vi "DOTNET - Network Ping v2.0.vi"(0 "IP/Address":string="127.0.0.1", 5 "SetSize":i32=32, 7 "timeout":i32=100, 11 "error in (no error)":errorcluster) -> (4 "Status":i32(ring) items=["Success"=0, "DestinationNetworkUnreachable"=11002, "DestinationHostUnreachable"=11003, "DestinationProhibited, DestinationProtocolUnreachable"=11004, "DestinationPortUnreachable"=11005, "NoResources"=11006, "BadOption"=11007, "HardwareError"=11008, "PacketTooBig"=11009, "TimedOut"=11010, "BadRoute"=11012, "TtlExpired"=11013, "TtlReassemblyTimeExceeded"=11014, "ParameterProblem"=11015, "SourceQuench"=11016, "BadDestination"=11018, "DestinationUnreachable"=11040, "TimeExceeded"=11041, "BadHeader"=11042, "UnrecognizedNextHeader"=11043, "IcmpError"=11044, "DestinationScopeMismatch"=11045, "Unknown"=-1], 6 "RoundtripTime":i64, 8 "found":bool, 15 "error out":errorcluster)   [LabVIEW 2020]
panel:
  out "Horizontal Graduated Bar":u8(slide) scale=0.0..30.0
  out "IP Adress":string
  # "Waiting for Kollmorgen Servo"
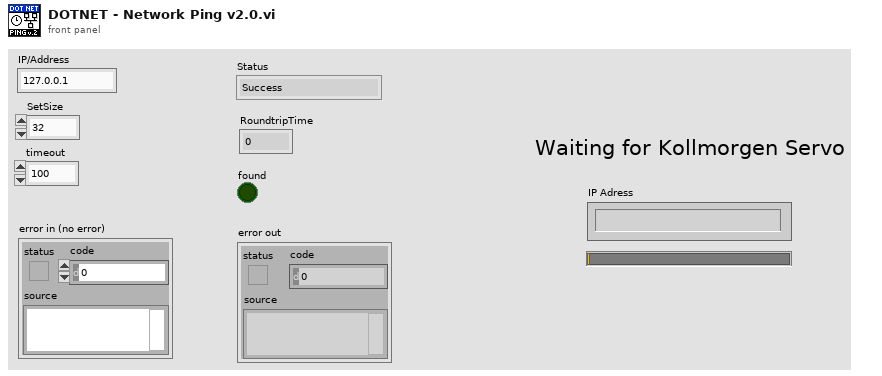
[diagram p1: front panel]
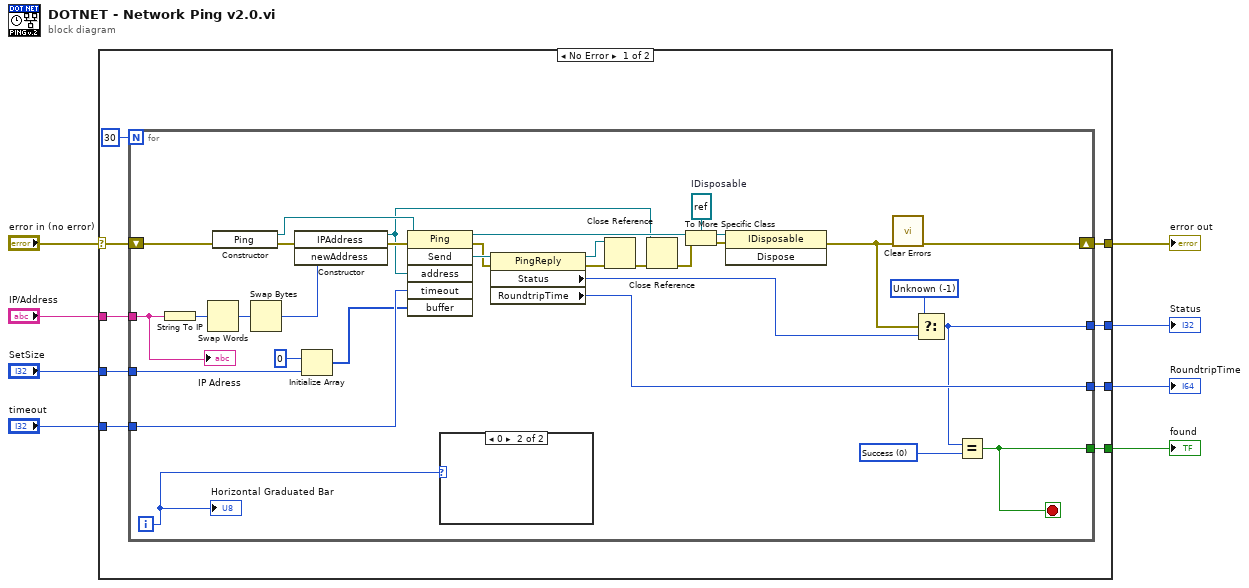
[diagram p0: block diagram]
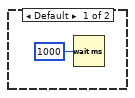
[diagram p2: hidden frame]
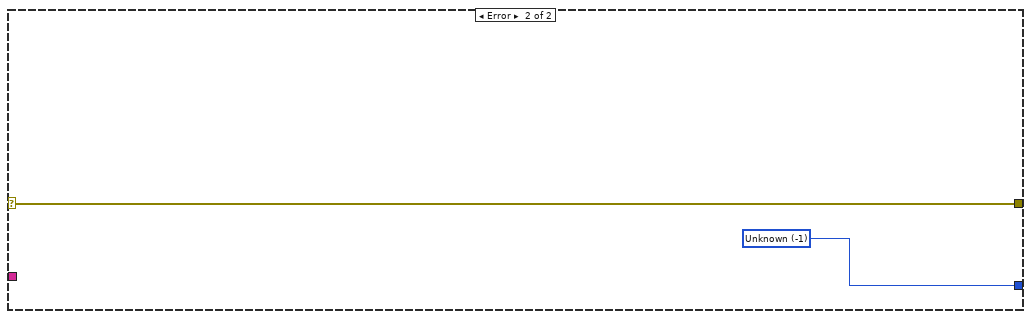
[diagram p3: hidden frame]
diagram:
  n1 = case shown="No Error" "error in (no error)" {
    selector: "error in (no error)" -> [w12 w52]
    tunnel: "IP/Address" -> [w17 _]
    tunnel: "timeout" -> [w16 _]
    tunnel: "SetSize" -> [w15 _]
    tunnel: [w11 w51] -> w5
    tunnel: [w14 _] -> w4
    tunnel: [w13 w52] -> w3
    tunnel: [w10 _] -> w1
    frame No Error {
      n2 = for {
        N: 30 -> [_]
        tunnel: w17 -> [w19]
        tunnel: w16 -> [w49]
        tunnel: w15 -> [w48]
        tunnel: [w47] -> w14
        tunnel: [w23] -> w11
        tunnel: [w20] -> w10
        shift-right: [w46] -> w13
        shift-left: w12 -> [w26]
        i -> [w18]
        stop <- w20 stop-if-true
        w22 = 0 items=["Success"=0, "DestinationNetworkUnreachable"=11002, "DestinationHostUnreachable"=11003, "DestinationProhibited, DestinationProtocolUnreachable"=11004, "DestinationPortUnreachable"=11005, "NoResources"=11006, "BadOption"=11007, "HardwareError"=11008, "PacketTooBig"=11009, "TimedOut"=11010, "BadRoute"=11012, "TtlExpired"=11013, "TtlReassemblyTimeExceeded"=11014, "ParameterProblem"=11015, "SourceQuench"=11016, "BadDestination"=11018, "DestinationUnreachable"=11040, "TimeExceeded"=11041, "BadHeader"=11042, "UnrecognizedNextHeader"=11043, "IcmpError"=11044, "DestinationScopeMismatch"=11045, "Unknown"=-1] ("Status")
        w24 = -1 items=["Success"=0, "DestinationNetworkUnreachable"=11002, "DestinationHostUnreachable"=11003, "DestinationProhibited, DestinationProtocolUnreachable"=11004, "DestinationPortUnreachable"=11005, "NoResources"=11006, "BadOption"=11007, "HardwareError"=11008, "PacketTooBig"=11009, "TimedOut"=11010, "BadRoute"=11012, "TtlExpired"=11013, "TtlReassemblyTimeExceeded"=11014, "ParameterProblem"=11015, "SourceQuench"=11016, "BadDestination"=11018, "DestinationUnreachable"=11040, "TimeExceeded"=11041, "BadHeader"=11042, "UnrecognizedNextHeader"=11043, "IcmpError"=11044, "DestinationScopeMismatch"=11045, "Unknown"=-1] ("Status")
        w34 = refnum<k24> refnum  # IDisposable
        n3 = String To IP(1:w19) -> (0:w38:u32)
        n4 = Swap Words(1:w38) -> (0:w36:u32)
        n5 = constructor class="Ping"(error in=w26) -> (reference out=w43:refnum<k24>, error out=w40:errorcluster)  [unwired: 2 in, 1 out]
        n6 = Swap Bytes(anything=w36) -> (byte swapped=w37:u32)
        n7 = constructor class="IPAddress"(error in=w40, "newAddress"=w37) -> (reference out=w30:refnum<k24>, error out=w39:errorcluster)  [unwired: 2 in, 2 out]
        n8 = Initialize Array(u8 0, w48) -> (w42:u8[])
        n9 = invoke class="Ping" method="Send"(reference=w43, error in=w39, "address"=w30, "timeout"=w49, "buffer"=w42) -> (reference out=w35:refnum<k24>, error out=w44:errorcluster, "Send"=w45:refnum<k24>)  [unwired: 1 in, 3 out]
        n10 = case shown="0" w18 {
          frame Default {
            n11 = Wait (ms)(milliseconds to wait=u32 1000) -> ()  [unwired: 1 out]
          }
          frame 0 {
          }
        }
        n12 = property class="PingReply"(reference=w45, error in=w44) -> (reference out=w33:refnum<k24>, error out=w32:errorcluster, "Status"=w25:i32, "RoundtripTime"=w47:i64)
        n13 = Close Reference(reference=w33, error in (no error)=w32) -> (error out=w31:errorcluster)
        n14 = Close Reference(reference=w30, error in (no error)=w31) -> (error out=w29:errorcluster)
        n15 = To More Specific Class(target class=w34, reference=w35, error in=w29) -> (specific class reference=w28:refnum<k24>, error out=w27:errorcluster)
        n16 = invoke class="IDisposable" method="Dispose"(reference=w28, error in=w27) -> (error out=w21:errorcluster)  [unwired: 1 in, 2 out]
        n17 = call <vilib>:"Clear Errors.vi"("error in (no error)"=w21) -> ("error out"=w46:errorcluster)  [unwired: 5 in, 1 out]
        n18 = Select(t=w24, s=w21, f=w25) -> (s? t:f=w23:i32)
        n19 = Equal?(x=w23, y=w22) -> (x = y?=w20:bool)
        "IP Adress" <- w19
        "Horizontal Graduated Bar" <- w18
      }
    }
    frame Error {
      w51 = -1 items=["Success"=0, "DestinationNetworkUnreachable"=11002, "DestinationHostUnreachable"=11003, "DestinationProhibited, DestinationProtocolUnreachable"=11004, "DestinationPortUnreachable"=11005, "NoResources"=11006, "BadOption"=11007, "HardwareError"=11008, "PacketTooBig"=11009, "TimedOut"=11010, "BadRoute"=11012, "TtlExpired"=11013, "TtlReassemblyTimeExceeded"=11014, "ParameterProblem"=11015, "SourceQuench"=11016, "BadDestination"=11018, "DestinationUnreachable"=11040, "TimeExceeded"=11041, "BadHeader"=11042, "UnrecognizedNextHeader"=11043, "IcmpError"=11044, "DestinationScopeMismatch"=11045, "Unknown"=-1] ("Status")
    }
  }
  "RoundtripTime" <- w4
  "error out" <- w3
  "Status" <- w5
  "found" <- w1
